vi "RT_ShVariables.vi"   [LabVIEW 2019]
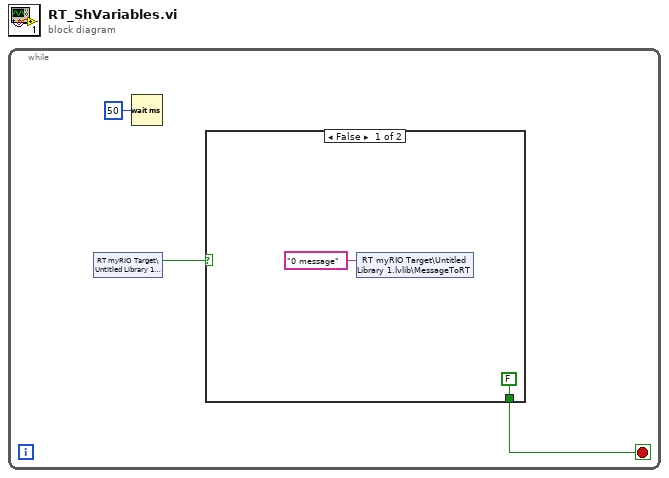
[diagram p0: block diagram]
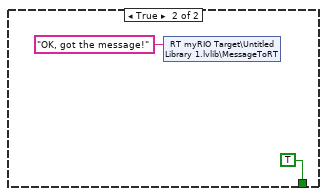
[diagram p2: hidden frame]
diagram:
  n1 = while {
    stop <- w1 stop-if-true
    n2 = shared-variable "RT myRIO Target\\Untitled Library 1.lvlib\\Stop"() -> (w3:bool)  [unwired: 1 in, 1 out]
    n3 = Wait (ms)(milliseconds to wait=u32 50) -> ()  [unwired: 1 out]
    n4 = case shown="False" w3 {
      tunnel: [FALSE TRUE] -> w1
      frame False {
        n5 = shared-variable "RT myRIO Target\\Untitled Library 1.lvlib\\MessageToRT"("0 message" ("MessageToRT")) -> ()  [unwired: 1 in, 1 out]
      }
      frame True {
        n6 = shared-variable "RT myRIO Target\\Untitled Library 1.lvlib\\MessageToRT"("OK, got the message!" ("MessageToRT")) -> ()  [unwired: 1 in, 1 out]
      }
    }
  }
